vi "Write_register_cmd.vi"(7 "Fifo-mode En":bool, 8 "Arty-7 Error In":errorcluster, 9 "Data Array":u8[](array[numeric]), 10 "WrReg Addr":u8 format="%b", 11 "Arty-7 VISA In":refnum<visa-resource-name>) -> (0 "Arty-7 Error out":errorcluster, 1 "WrReg Status":string, 2 "WrReg Done":bool, 3 "Arty-7 VISA out":refnum<visa-resource-name>)   [LabVIEW 2019]
uses:
  <vilib>/Utility/error.llb/DialogType.ctl
  Board_Global_Var.vi
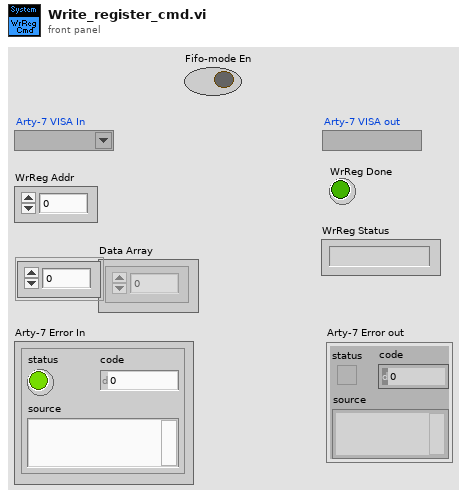
[diagram p1: front panel]
types:
  T1 = typedef "DialogType.ctl" = u16
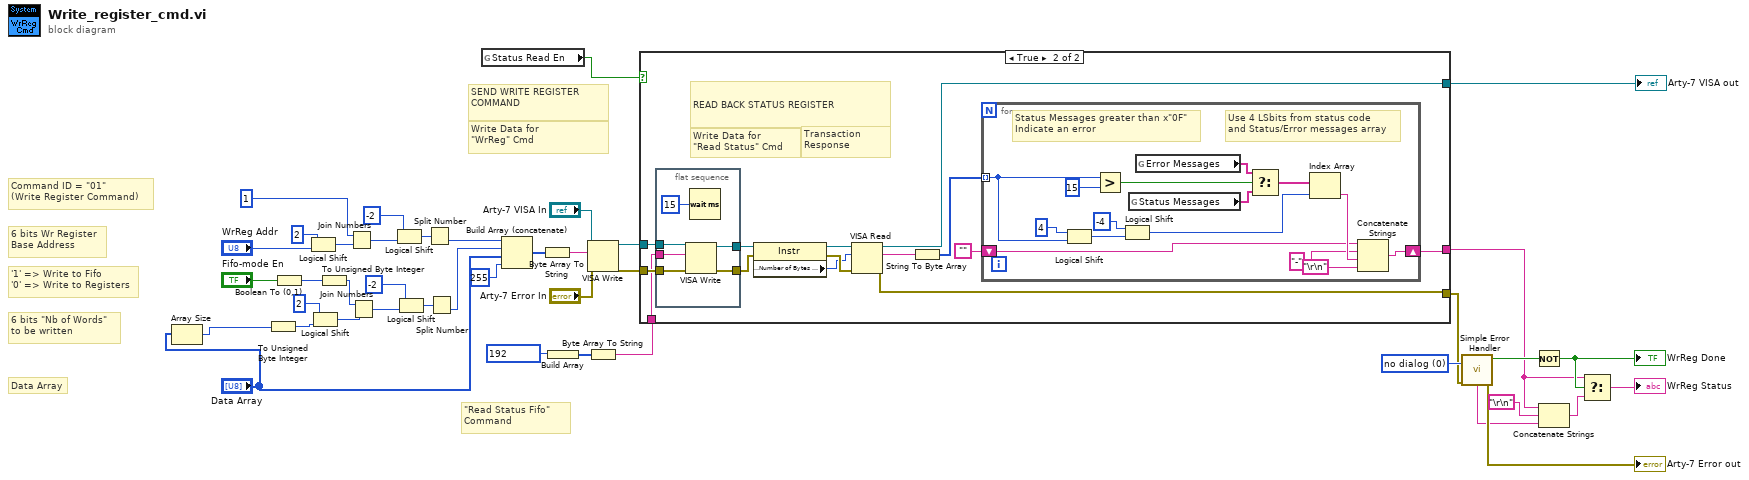
[diagram p0: block diagram]
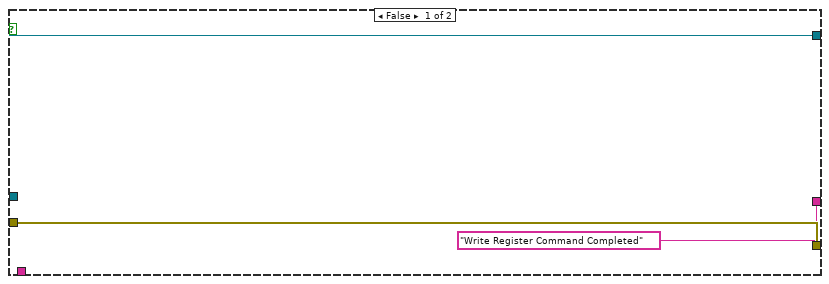
[diagram p2: hidden frame]
diagram:
  w8 = T1 0 items=["no dialog", "OK message", "continue or stop message", "OK message + warnings", "continue/stop + warnings"] ("type of dialog (OK msg:1)")
  # "SEND WRITE REGISTER\nCOMMAND"
  # "Write Data for \n\"WrReg\" Cmd"
  # "\"Read Status Fifo\" \nCommand"
  # "Data Array"
  # "'1' => Write to Fifo\n'0' => Write to Registers"
  # "6 bits \"Nb of Words\"\nto be written"
  # "6 bits Wr Register \nBase Address"
  # "Command ID = \"01\" \n(Write Register Command)"
  n1 = Array Size(array="Data Array") -> (size(s)=w19:i32)
  n2 = To Unsigned Byte Integer(number=w19) -> (unsigned 8bit integer=w42:u8)
  n3 = Boolean To (0,1)(Boolean="Fifo-mode En") -> (0, 1=w37:i16)
  n4 = Logical Shift(y=i16 2, x="WrReg Addr") -> (x << y=w25:u8)
  n5 = Logical Shift(y=i16 2, x=w42) -> (x << y=w32:u8)
  n6 = To Unsigned Byte Integer(number=w37) -> (unsigned 8bit integer=w38:u8)
  n7 = Join Numbers(hi=u8 1, lo=w25) -> ((hi.lo)=w24:u16)
  n8 = Join Numbers(hi=w38, lo=w32) -> ((hi.lo)=w33:u16)
  n9 = Logical Shift(y=i16 -2, x=w24) -> (x << y=w28:u16)
  n10 = Logical Shift(y=i16 -2, x=w33) -> (x << y=w30:u16)
  n11 = Split Number(x=w28) -> (lo(x)=w29:u8)  [unwired: 1 out]
  n12 = Split Number(x=w30) -> (lo(x)=w35:u8)  [unwired: 1 out]
  n13 = global read "Board_Global_Var.vi" "Status Read En"() -> (w1:bool)
  n14 = Build Array (concatenate)(w29, w35, "Data Array", u8 255 ("WrReg Addr 2")) -> (w40:u8[])
  n15 = Byte Array To String(unsigned byte array=w40) -> (string=w39:string)
  n16 = Build Array(u8 192) -> (w12:u8[])
  n17 = VISA Write(VISA resource name="Arty-7 VISA In", write buffer=w39, error in (no error)="Arty-7 Error In") -> (VISA resource name out=w17:refnum<visa-resource-name>, error out=w16:errorcluster)  [unwired: 1 out]
  n18 = Byte Array To String(unsigned byte array=w12) -> (string=w10:string)
  n19 = case shown="True" w1 {
    tunnel: w17 -> [w44 w59]
    tunnel: w16 -> [w45 w58]
    tunnel: [w44 w57] -> w15
    tunnel: w10 -> [_ w56]
    tunnel: [w45 w55] -> w7
    tunnel: ["Write Register Command Completed" w53] -> w6
    frame False {
    }
    frame True {
      # "READ BACK STATUS REGISTER"
      # "Write Data for \n\"Read Status\" Cmd"
      # "Transaction \nResponse"
      n20 = flat-sequence {
        tunnel: w59 -> [w65]
        tunnel: w58 -> [w64]
        tunnel: w56 -> [w63]
        tunnel: [w62] -> w52
        tunnel: [w61] -> w51
        frame #0 {
          n21 = VISA Write(VISA resource name=w65, write buffer=w63, error in (no error)=w64) -> (VISA resource name out=w62:refnum<visa-resource-name>, error out=w61:errorcluster)  [unwired: 1 out]
          n22 = Wait (ms)(milliseconds to wait=u32 15) -> ()  [unwired: 1 out]
        }
      }
      n23 = property class="Instr"(reference=w52, error in=w51) -> (reference out=w50:refnum<visa-resource-name>, error out=w49:errorcluster, "Serial Settings:Number of Bytes at Serial Port"=w48:u32)
      n24 = VISA Read(VISA resource name=w50, byte count=w48, error in (no error)=w49) -> (VISA resource name out=w57:refnum<visa-resource-name>, read buffer=w54:string, error out=w55:errorcluster)  [unwired: 1 out]
      n25 = String To Byte Array(string=w54) -> (unsigned byte array=w47:u8[])
      n26 = for {
        tunnel: w47 -> [w70] mode=indexing
        shift-right: [w69] -> w53
        shift-left: "" -> [w68]
        # "Use 4 LSbits from status code \nand Status/Error messages array"
        # "Status Messages greater than x\"0F\"\nIndicate an error"
        n27 = Logical Shift(y=i16 4, x=w70) -> (x << y=w73:u8)
        n28 = Greater?(x=w70, y=u8 15) -> (0:w76:bool)
        n29 = Logical Shift(y=i16 -4, x=w73) -> (x << y=w74:u8)
        n30 = global read "Board_Global_Var.vi" "Status Messages"() -> (w77:string[])
        n31 = global read "Board_Global_Var.vi" "Error Messages"() -> (w78:string[])
        n32 = Select(t=w78, s=w76, f=w77) -> (s? t:f=w79:string[])
        n33 = Index Array(array=w79, index=w74) -> (element=w71:string)
        n34 = Concatenate Strings(w68, "-" ("string"), w71, "\r\n") -> (w69:string)
      }
    }
  }
  "Arty-7 VISA out" <- w15
  n35 = call <vilib>:"Simple Error Handler.vi"("type of dialog (OK msg:1)"=w8, "error in (no error)"=w7) -> ("error?"=w9:bool, "error out"=→"Arty-7 Error out":errorcluster, "message"=w4:string)  [unwired: 3 in, 2 out]
  n36 = Not(x=w9) -> (.not. x?=w14:bool)
  "WrReg Done" <- w14
  n37 = Concatenate Strings(w6, "\r\n", w4) -> (w3:string)
  n38 = Select(t=w6, s=w14, f=w3) -> (s? t:f=→"WrReg Status":string)
